vi "digital write all.vi"(8 "error in (no error)":errorcluster, 10 "data":bool[](array[boolean]), 11 "USB-6000 in":refnum<class "USB-6000.lvclass">) -> (0 "error out":errorcluster, 3 "USB-6000 out":refnum<class "USB-6000.lvclass">)   [LabVIEW 2025, in "USB IO.lvlib" / "USB-6000.lvclass"]
uses:
  USB-6000.lvclass
  USB-6000.lvclass/USB-6000.ctl
  <vilib>/DAQmx/write.llb/DAQmx Write (Digital 1D Bool 1Chan 1Samp).vi
  <vilib>/DAQmx/miscellaneous.llb/DAQmx Fill In Error Info.vi
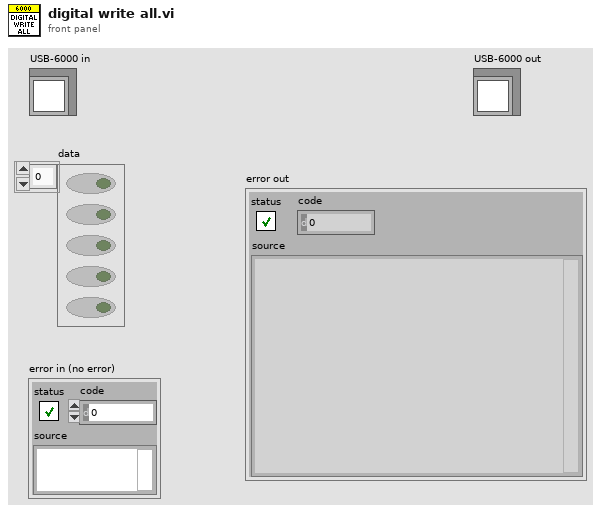
[diagram p1: front panel]
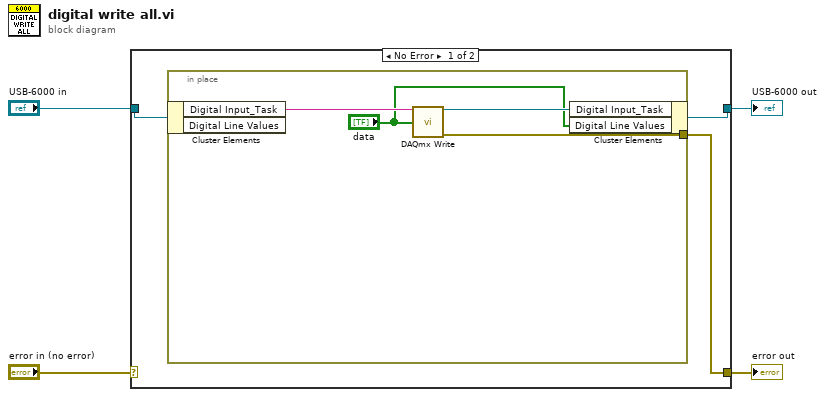
[diagram p0: block diagram]
diagram:
  n1 = case shown="No Error" "error in (no error)" {
    selector: "error in (no error)" -> [_ w13]
    tunnel: [w5 w13] -> w3
    tunnel: [w6 w12] -> w1
    tunnel: "USB-6000 in" -> [w7 w12]
    frame No Error {
      n2 = in-place {
        in-place-border: [w9] -> w5
        n3 = in-place-cluster #1(w7) -> ("Digital Input_Task"=w10:string)  [unwired: 1 out]
        n4 = call-poly <vilib>:"DAQmx Write.vi"("task/channels in"=w10, "data"="data") -> ("task out"=w11:refnum<k21>, "error out"=w9:errorcluster)  [unwired: 11 in, 1 out]
        n5 = in-place-cluster #1("Digital Input_Task"=w11, "Digital Line Values"="data") -> (w6:refnum<class "USB-6000.lvclass">)
      }
    }
    frame Error {
    }
  }
  "error out" <- w3
  "USB-6000 out" <- w1
